vi "LabVIEW to JSON.vi"(8 "error in (no error)":errorcluster, 10 "Data":dbl) -> (0 "error out":errorcluster, 3 "JSON out":refnum<class "JSON Value.lvclass">)   [LabVIEW 2016, in "JSON Value.lvclass"]
uses:
  JSON Value.lvclass
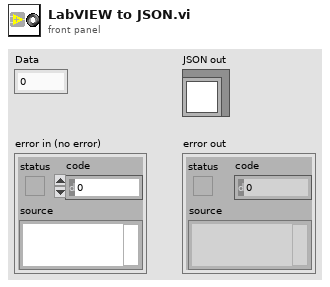
[diagram p1: front panel]
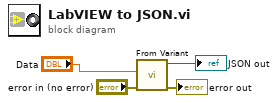
[diagram p0: block diagram]
diagram:
  n1 = call "From Variant.vi"("error in (no error)"="error in (no error)", "Variant"="Data") -> ("error out"=→"error out":errorcluster, "JSON out"=→"JSON out":refnum<class "JSON Value.lvclass">)  [unwired: 8 in]
